vi "EAGLE RT Simulator.vi"() -> ()   [LabVIEW 2015]
panel:
  in  "stop":bool
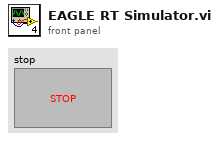
[diagram p1: front panel]
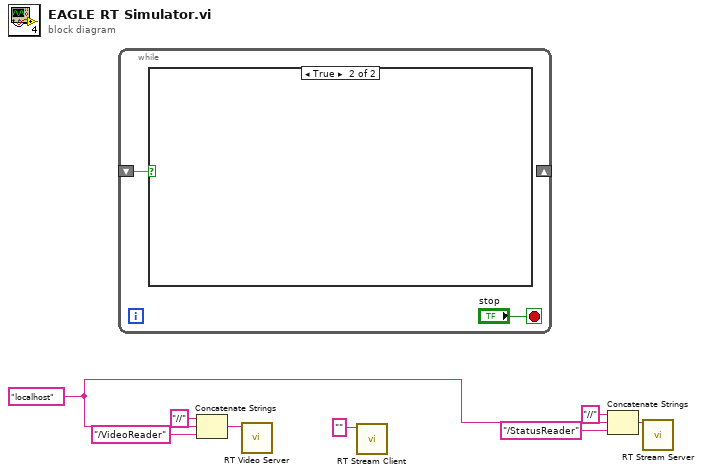
[diagram p0: block diagram]
diagram:
  w1 = "localhost" ("HostIP")
  n1 = while {
    shift-right: _ -> [_]
    shift-left: _ -> [w9]
    stop <- "stop" stop-if-true
    n2 = case shown="True" w9 {
      frame False {
      }
      frame True {
      }
    }
  }
  n3 = Concatenate Strings("//" ("string"), w1, "/VideoReader" ("reader url")) -> (w6:string)
  n4 = call "RT Video Server.vi"("reader url"=w6) -> ()  [unwired: 11 in]
  n5 = call "RT Stream Client.vi"("Writer url"="") -> ()  [unwired: 11 in]
  n6 = Concatenate Strings("//" ("string"), w1, "/StatusReader" ("reader url")) -> (w3:string)
  n7 = call "RT Stream Server.vi"("reader url"=w3) -> ()  [unwired: 11 in]
